vi "ezAFM Practice 1.7.vi"() -> ()   [LabVIEW 2015]
uses:
  D:/LabVIEW for ezAFM/LV-PGC 2019-05a/Special Equipment/ezAFM/NMI Integration Code/ezCommander.dll
  LabVIEW for ezAFM/LV-PGC 2019-05a/Special Equipment/ezAFM/NMI Integration Code/ezCommander.dll
  <vilib>/userdefined/High Color/IMAQdx.ctl
  LabVIEW for ezAFM/LV-PGC 2019-05a/Universal vi's/Global Variables/Globals-EasyAFM.vi
  Globals.vi
  <vilib>/vision/driver/NI_Vision_Acquisition_Software.lvlib
panel:
  out "Index":dbl
  out "Direction":dbl
  out "Searching":bool
  out "Crosshair Found?":bool
  in  "Search":bool
  out "Total Steps":dbl
  out "Current Steps":dbl
  in  "Camera":enum32{"ezAFM Camera"}(tab)
  out "ezAFM Camera":T1(plugin-control)
  in  "Connection to Scan":string
  in  "Enable Automatic \nRepositioning":bool
  out "Imaging Status":string
  out "Automated Imaging":bool
  in  "Main Menu":enum32{"Navigation", "Scanning"}(tab)
  in  "APPROACH":bool
  in  "RETRACT":bool
  in  "Step Size":dbl
  in  "Angle":dbl
  in  "THETA":bool
  in  "MOVE2CROSSHAIR":bool
  in  "Current Crosshair":string(combo)="00 | 01"
  in  "Target Crosshair":string(combo)="00 | 01"
  in  "Motor Speed":u16(ring)=30000 items=["SLOW"=3300, "MEDIUM"=30000, "FAST"=65000]
  in  "Navigation Buttons":T2
  in  "SEARCH":bool
  in  "Image Resolution":u16(ring)=256 items=["32"=32, "64"=64, "128"=128, "256"=256, "512"=512, "1024"=1024, "2048"=2048]
  in  "SELECT CONNECTIONS":bool
  in  "Initialize Automated Imaging":bool
  out "Connections":string[](array[string])
  out "Sequence":string[](array[string])
  in  "Indicators":enum32{"Indicators"}(tab)
  out "XYZ Motor Position":dbl[](array[numeric]) format="%#_4f"
  out "ezAFM Status":dbl
  out "Approaching":bool
  out "ezAFM Connected":bool
  out "Retracting":bool
  out "Scan":bool caption="Scanning"
  out "Tip Approached?":bool
  in  "RESET":bool
  out "XY Position":dbl[](array[numeric])
  in  "QUIT":bool
  # "Use Arrow Keys to manually\nmove the XY Motor"
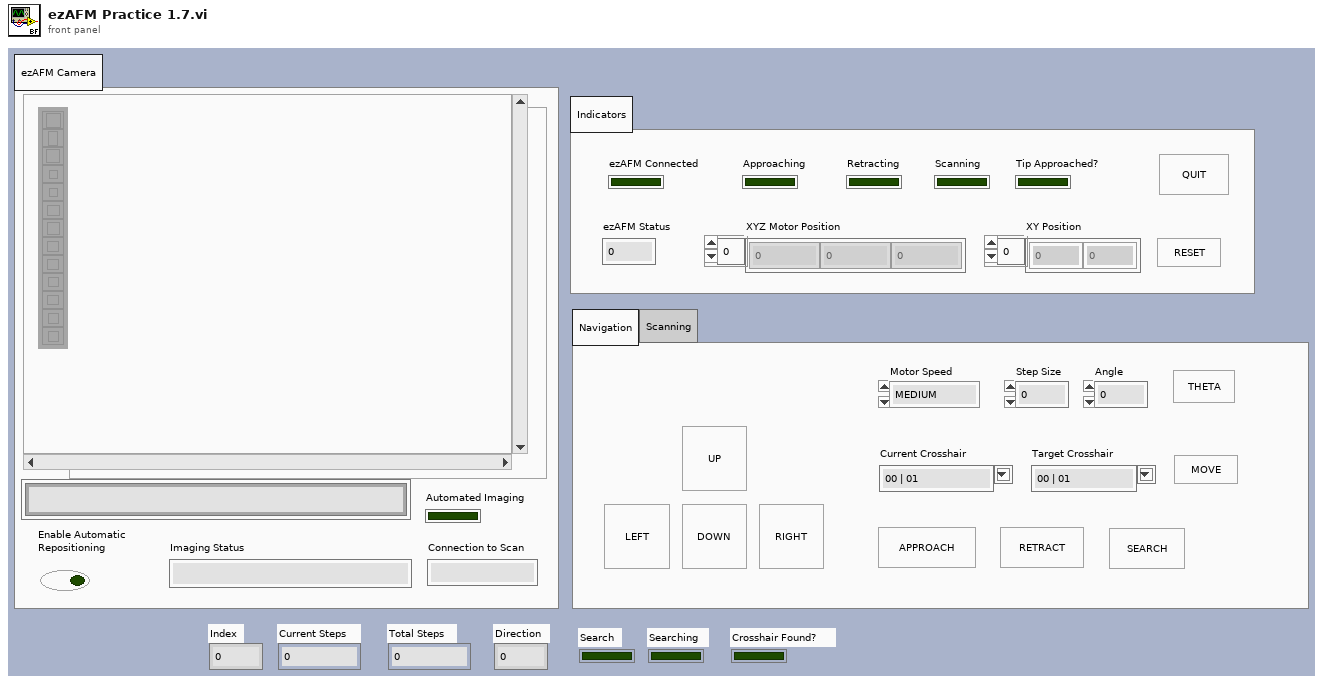
[diagram p1: front panel]
types:
  T1 = typedef "IMAQ Image.ctl" = refnum<image>
  T2 = cluster{"UP":bool, "DOWN":bool, "LEFT":bool, "RIGHT":bool}
  T3 = typedef "IMAQdx.ctl" = refnum<k21>
  T4 = typedef "Image Type" = u32
  T5 = typedef "eventvkey.ctl" = enum16{"ASCII", "Enter", "Return", "Shift", "Ctrl", "Alt", "Cmd", "Opt", "Caps", "NumLock", "Clear", "Break", "Up", "Down", "Left", "Right", "Insert", "Delete", "Home", "End", "PageUp", "PageDown", "Escape", "Help", "Pause", "ScrollLock", "F1", "F2", "F3", "F4", "F5", "F6", "F7", "F8", "F9", "F10", "F11", "F12", "F13", "F14", "F15", "F16", "F17", "F18", "F19", "F20", "F21", "F22", "F23", "F24", "Play", "VolumeUp", "VolumeDown", "Mute", "Two Byte Char"}
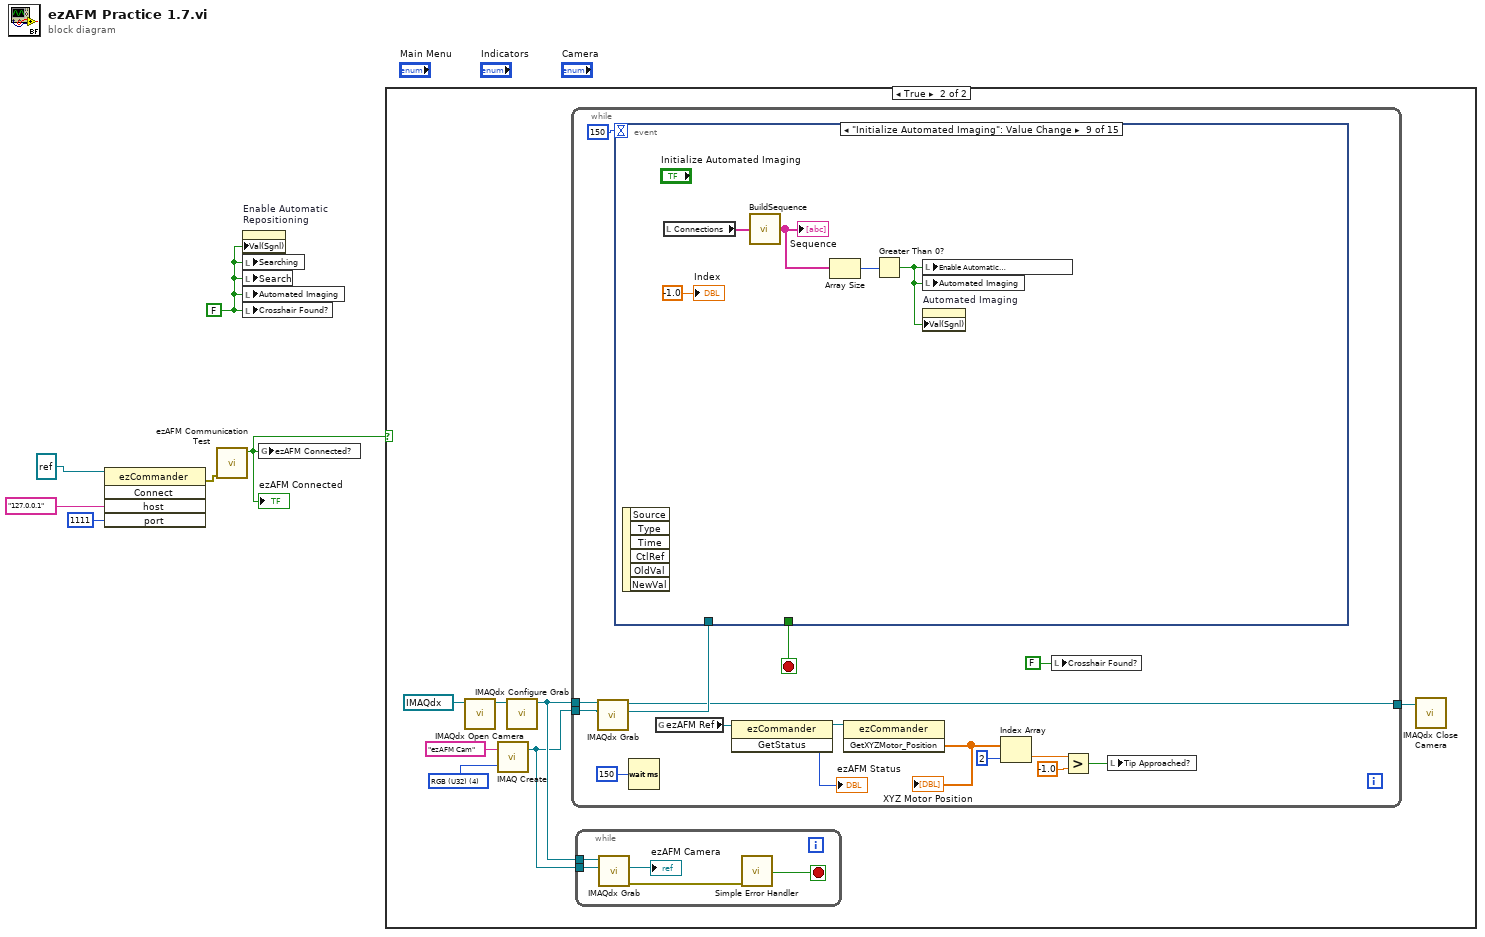
[diagram p0: block diagram]
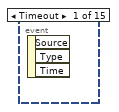
[diagram p3: hidden frame]
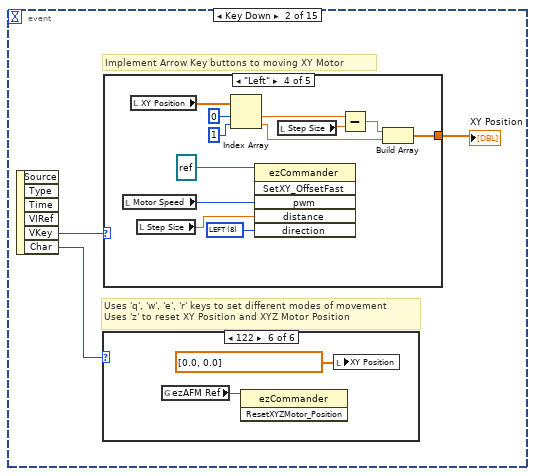
[diagram p4: hidden frame]
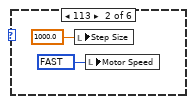
[diagram p6: hidden frame]
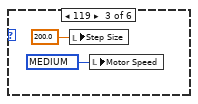
[diagram p7: hidden frame]
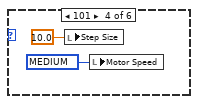
[diagram p8: hidden frame]
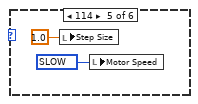
[diagram p9: hidden frame]
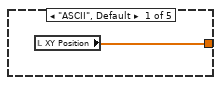
[diagram p10: hidden frame]
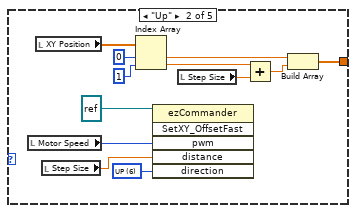
[diagram p11: hidden frame]
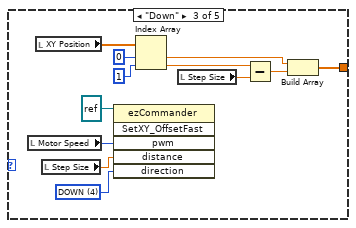
[diagram p12: hidden frame]
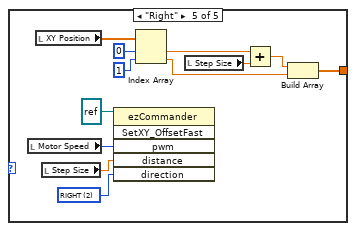
[diagram p13: hidden frame]
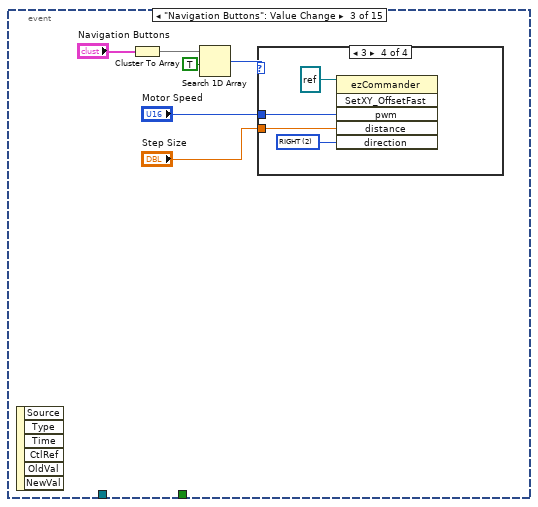
[diagram p14: hidden frame]
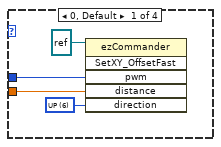
[diagram p15: hidden frame]
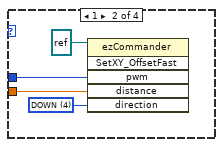
[diagram p16: hidden frame]
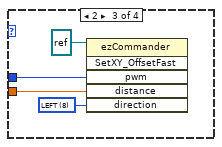
[diagram p17: hidden frame]
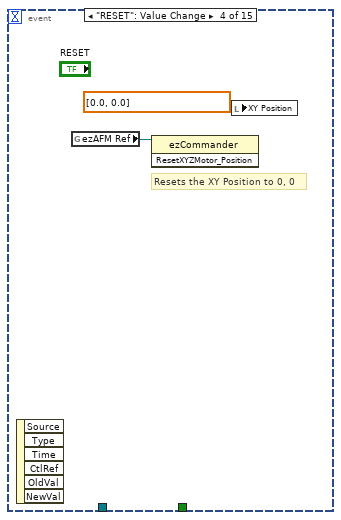
[diagram p18: hidden frame]
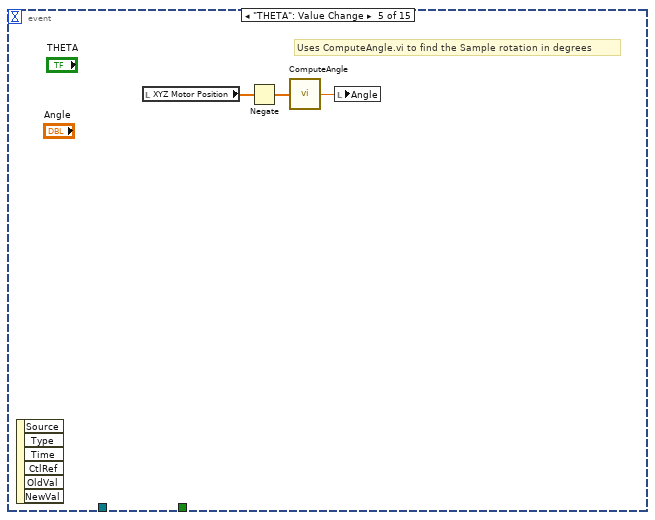
[diagram p19: hidden frame]
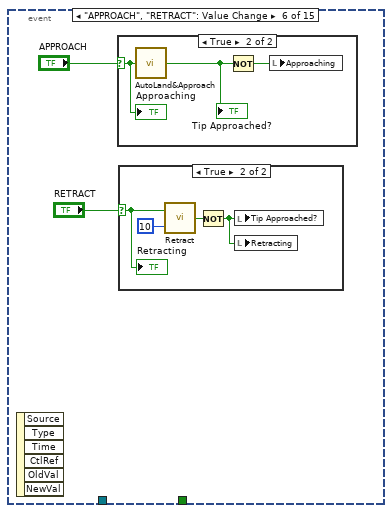
[diagram p20: hidden frame]
diagram:
  w1 = FALSE ("Automated Imaging")
  n1 = invoke class="ezCommander" method="Connect"(reference=refnum<k24> refnum ("ezAFM Ref"), "host"="127.0.0.1", "port"=1111) -> (error out=w5:errorcluster)  [unwired: 2 in, 4 out]
  n2 = call "ezAFM Communication Test.vi"("error in"=w5) -> ("ezAFM COM status"=w2:bool)  [unwired: 3 in, 3 out]
  "ezAFM Connected" <- w2
  n3 = property on="Enable Automatic \nRepositioning" class="Bool (strict)"("Val(Sgnl)"=w1) -> ()  [unwired: 2 in, 2 out]
  n4 = local write "Searching"(w1) -> ()
  n5 = local write "Search"(w1) -> ()
  n6 = local write "Automated Imaging"(w1) -> ()
  n7 = local write "Crosshair Found?"(w1) -> ()
  n8 = global write "Globals.vi" "ezAFM Connected?"(w2) -> ()
  n9 = case shown="True" w2 {
    frame False {
    }
    frame True {
      w10 = T4 4 items=["Grayscale (U8)", "Grayscale (I16)", "Grayscale (SGL)", "Complex (CSG)", "RGB (U32)", "HSL (U32)", "RGB (U64)", "Grayscale (U16)"] ("Image Type")
      n10 = call <vilib>:"IMAQdx Open Camera.vi"("Session In"=T3 "cam5") -> ("Session Out"=w11:T3)  [unwired: 9 in, 1 out]
      n11 = call "IMAQ Create"("Image Name"="ezAFM Cam", "Image Type"=w10) -> ("New Image"=w8:T1)  [unwired: 3 in, 1 out]
      n12 = call <vilib>:"IMAQdx Configure Grab.vi"("Session In"=w11) -> ("Session Out"=w9:T3)  [unwired: 9 in, 1 out]
      n13 = while {
        tunnel: w9 -> [w24]
        tunnel: w8 -> [w23]
        tunnel: [w21] -> w7
        stop <- w20 stop-if-true
        n14 = call <vilib>:"IMAQdx Grab.vi"("Image In"=w23, "Session In"=w24) -> ("Image Out"=w22:T1, "Session Out"=w21:T3)  [unwired: 2 in, 6 out]
        n15 = event shown="[8] \"Initialize Automated Imaging\": Value Change" {
          selector: _ -> [_ _ _ _ _ _ _ _ _ _ _ _ _ _ _]
          dyn-events: _ -> [_ _ _ _ _ _ _ _ _ _ _ _ _ _ _]
          timeout: 150 -> [_ _ _ _ _ _ _ _ _ _ _ _ _ _ _]
          tunnel: [_ _ _ _ _ _ _ _ _ _ _ _ _ _ "QUIT"] -> w20
          tunnel: w22 -> [_ _ _ _ _ _ _ _ _ _ _ _ w188 _ _]
          event Timeout {
            n16 = event-data() -> ()  [unwired: 1 in, 3 out]
          }
          event Key Down {
            # "Uses 'q', 'w', 'e', 'r' keys to set different modes of movement\nUses 'z' to reset XY Position and XYZ Motor Position"
            # "Implement Arrow Key buttons to moving XY Motor"
            n17 = event-data() -> ("VKey"=w35:T5, "Char"=w36:i16)  [unwired: 1 in, 4 out]
            n18 = case shown="122" w36 {
              frame 0, Default {
              }
              frame 113 {
                w38 = u16 65000 items=["SLOW"=3300, "MEDIUM"=30000, "FAST"=65000] ("Motor Speed")
                n19 = local write "Step Size"(1000.0 ("Step Size")) -> ()
                n20 = local write "Motor Speed"(w38) -> ()
              }
              frame 119 {
                w40 = u16 30000 items=["SLOW"=3300, "MEDIUM"=30000, "FAST"=65000] ("Motor Speed")
                n21 = local write "Step Size"(200.0 ("Step Size")) -> ()
                n22 = local write "Motor Speed"(w40) -> ()
              }
              frame 101 {
                w42 = u16 30000 items=["SLOW"=3300, "MEDIUM"=30000, "FAST"=65000] ("Motor Speed")
                n23 = local write "Step Size"(10.0 ("Step Size")) -> ()
                n24 = local write "Motor Speed"(w42) -> ()
              }
              frame 114 {
                w44 = u16 3300 items=["SLOW"=3300, "MEDIUM"=30000, "FAST"=65000] ("Motor Speed")
                n25 = local write "Step Size"(1.0 ("Step Size")) -> ()
                n26 = local write "Motor Speed"(w44) -> ()
              }
              frame 122 {
                n27 = global read "Globals-EasyAFM.vi" "ezAFM Ref"() -> (w46:refnum<k24>)
                n28 = invoke class="ezCommander" method="ResetXYZMotor_Position"(reference=w46) -> ()  [unwired: 2 in, 3 out]
                n29 = local write "XY Position"(dbl[] [0.0, 0.0] ("XY Position")) -> ()
              }
            }
            n30 = case shown="\"Left\"" w35 {
              tunnel: [w48 w50 w61 w73 w85] -> w37
              frame "ASCII", Default {
                n31 = local read "XY Position"() -> (w48:dbl[])
              }
              frame "Up" {
                w59 = u16 6 items=["UP"=6, "DOWN"=4, "LEFT"=8, "RIGHT"=2]
                n32 = local read "Motor Speed"() -> (w58:u16)
                n33 = local read "XY Position"() -> (w56:dbl[])
                n34 = local read "Step Size"() -> (w57:dbl)
                n35 = Index Array(array=w56, index #1=0 ("index"), index #2=1 ("index")) -> (element #1=w52:dbl, element #2=w49:dbl)
                n36 = invoke class="ezCommander" method="SetXY_OffsetFast"(reference=refnum<k24> refnum ("ezAFM Ref"), "pwm"=w58, "distance"=w57, "direction"=w59) -> ()  [unwired: 2 in, 6 out]
                n37 = local read "Step Size"() -> (w53:dbl)
                n38 = Add(x=w49, y=w53) -> (x+y=w51:dbl)
                n39 = Build Array(w52, w51) -> (w50:dbl[])
              }
              frame "Down" {
                w69 = u16 4 items=["UP"=6, "DOWN"=4, "LEFT"=8, "RIGHT"=2]
                n40 = local read "Motor Speed"() -> (w71:u16)
                n41 = local read "XY Position"() -> (w63:dbl[])
                n42 = local read "Step Size"() -> (w70:dbl)
                n43 = invoke class="ezCommander" method="SetXY_OffsetFast"(reference=refnum<k24> refnum ("ezAFM Ref"), "pwm"=w71, "distance"=w70, "direction"=w69) -> ()  [unwired: 2 in, 6 out]
                n44 = Index Array(array=w63, index #1=0 ("index"), index #2=1 ("index")) -> (element #1=w65:dbl, element #2=w66:dbl)
                n45 = local read "Step Size"() -> (w62:dbl)
                n46 = Subtract(x=w66, y=w62) -> (x-y=w64:dbl)
                n47 = Build Array(w65, w64) -> (w61:dbl[])
              }
              frame "Left" {
                w83 = u16 8 items=["UP"=6, "DOWN"=4, "LEFT"=8, "RIGHT"=2]
                n48 = local read "Motor Speed"() -> (w81:u16)
                n49 = local read "XY Position"() -> (w77:dbl[])
                n50 = local read "Step Size"() -> (w82:dbl)
                n51 = Index Array(array=w77, index #1=0 ("index"), index #2=1 ("index")) -> (element #1=w76:dbl, element #2=w74:dbl)
                n52 = invoke class="ezCommander" method="SetXY_OffsetFast"(reference=refnum<k24> refnum ("ezAFM Ref"), "pwm"=w81, "distance"=w82, "direction"=w83) -> ()  [unwired: 2 in, 6 out]
                n53 = local read "Step Size"() -> (w78:dbl)
                n54 = Subtract(x=w76, y=w78) -> (x-y=w75:dbl)
                n55 = Build Array(w75, w74) -> (w73:dbl[])
              }
              frame "Right" {
                w95 = u16 2 items=["UP"=6, "DOWN"=4, "LEFT"=8, "RIGHT"=2]
                n56 = local read "Motor Speed"() -> (w94:u16)
                n57 = local read "XY Position"() -> (w90:dbl[])
                n58 = local read "Step Size"() -> (w93:dbl)
                n59 = invoke class="ezCommander" method="SetXY_OffsetFast"(reference=refnum<k24> refnum ("ezAFM Ref"), "pwm"=w94, "distance"=w93, "direction"=w95) -> ()  [unwired: 2 in, 6 out]
                n60 = Index Array(array=w90, index #1=0 ("index"), index #2=1 ("index")) -> (element #1=w88:dbl, element #2=w86:dbl)
                n61 = local read "Step Size"() -> (w89:dbl)
                n62 = Add(x=w88, y=w89) -> (x+y=w87:dbl)
                n63 = Build Array(w87, w86) -> (w85:dbl[])
              }
            }
            "XY Position" <- w37
          }
          event "Navigation Buttons": Value Change {
            n64 = event-data() -> ()  [unwired: 1 in, 6 out]
            n65 = Cluster To Array(cluster="Navigation Buttons") -> (array=w101:bool[])
            n66 = Search 1D Array(1D array=w101, element=TRUE) -> (index of element=w99:i32)  [unwired: 1 in]
            n67 = case shown="3" w99 {
              tunnel: "Step Size" -> [w103 w108 w112 w116]
              tunnel: "Motor Speed" -> [w104 w107 w111 w115]
              frame 0, Default {
                w105 = u16 6 items=["UP"=6, "DOWN"=4, "LEFT"=8, "RIGHT"=2]
                n68 = invoke class="ezCommander" method="SetXY_OffsetFast"(reference=refnum<k24> refnum ("ezAFM Ref"), "pwm"=w104, "distance"=w103, "direction"=w105) -> ()  [unwired: 2 in, 6 out]
              }
              frame 1 {
                w109 = u16 4 items=["UP"=6, "DOWN"=4, "LEFT"=8, "RIGHT"=2]
                n69 = invoke class="ezCommander" method="SetXY_OffsetFast"(reference=refnum<k24> refnum ("ezAFM Ref"), "pwm"=w107, "distance"=w108, "direction"=w109) -> ()  [unwired: 2 in, 6 out]
              }
              frame 2 {
                w113 = u16 8 items=["UP"=6, "DOWN"=4, "LEFT"=8, "RIGHT"=2]
                n70 = invoke class="ezCommander" method="SetXY_OffsetFast"(reference=refnum<k24> refnum ("ezAFM Ref"), "pwm"=w111, "distance"=w112, "direction"=w113) -> ()  [unwired: 2 in, 6 out]
              }
              frame 3 {
                w117 = u16 2 items=["UP"=6, "DOWN"=4, "LEFT"=8, "RIGHT"=2]
                n71 = invoke class="ezCommander" method="SetXY_OffsetFast"(reference=refnum<k24> refnum ("ezAFM Ref"), "pwm"=w115, "distance"=w116, "direction"=w117) -> ()  [unwired: 2 in, 6 out]
              }
            }
          }
          event "RESET": Value Change {
            # "Resets the XY Position to 0, 0"
            n72 = event-data() -> ()  [unwired: 1 in, 6 out]
            n73 = global read "Globals-EasyAFM.vi" "ezAFM Ref"() -> (w119:refnum<k24>)
            n74 = invoke class="ezCommander" method="ResetXYZMotor_Position"(reference=w119) -> ()  [unwired: 2 in, 3 out]
            n75 = local write "XY Position"(dbl[] [0.0, 0.0] ("XY Position")) -> ()
          }
          event "THETA": Value Change {
            # "Uses ComputeAngle.vi to find the Sample rotation in degrees"
            n76 = event-data() -> ()  [unwired: 1 in, 6 out]
            n77 = local read "XYZ Motor Position"() -> (w122:dbl[])
            n78 = Negate(x=w122) -> (-x=w123:dbl[])
            n79 = call "ComputeAngle.vi"("XY Vector"=w123) -> ("Angle"=w121:dbl)
            n80 = local write "Angle"(w121) -> ()
          }
          event "APPROACH", "RETRACT": Value Change {
            n81 = event-data() -> ()  [unwired: 1 in, 6 out]
            n82 = case shown="True" "APPROACH" {
              selector: "APPROACH" -> [_ w131]
              frame False {
              }
              frame True {
                n83 = call "AutoLand&Approach.vi"("Approaching?"=w131) -> ("Finished?"=w130:bool)
                "Tip Approached?" <- w130
                n84 = Not(x=w130) -> (.not. x?=w132:bool)
                n85 = local write "Approaching"(w132) -> ()
                "Approaching" <- w131
              }
            }
            n86 = case shown="True" "RETRACT" {
              selector: "RETRACT" -> [_ w126]
              frame False {
              }
              frame True {
                n87 = call "Retract.vi"("Number of Cycles"=10, "Retracting?"=w126) -> ("Finished?"=w128:bool)
                n88 = Not(x=w128) -> (.not. x?=w127:bool)
                n89 = local write "Tip Approached?"(w127) -> ()
                n90 = local write "Retracting"(w127) -> ()
                "Retracting" <- w126
              }
            }
          }
          event "MOVE2CROSSHAIR": Value Change {
            w138 = u16 65000 items=["SLOW"=3300, "MEDIUM"=30000, "FAST"=65000] ("Motor Speed")
            # "XY Vector is in cartesian coordinates of the Oasis Camera\nUses Move2Device.vi to find the XY Vector between the Current Device and Target Device crosshairs\nInputs the XY Vector into Move2Vector.vi to command the XY Motor to move"
            n91 = event-data() -> ()  [unwired: 1 in, 6 out]
            n92 = call "GetCrosshairVector.vi"("Target Crosshair"="Target Crosshair", "Current Crosshair"="Current Crosshair") -> ("XY Vector"=w133:dbl[])  [unwired: 9 in]
            n93 = local read "Angle"() -> (w137:dbl)
            n94 = call "Move2Vector.vi"("Motor Speed"=w138, "Angle"=w137, "XY Vector"=w133) -> ("Finished?"=w136:bool)  [unwired: 8 in]
            n95 = case shown="True" w136 {
              frame False {
              }
              frame True {
                n96 = local read "Enable Automatic \nRepositioning"() -> (w141:bool)
                n97 = local read "Target Crosshair"() -> (w140:string)
                n98 = local write "MOVE2CROSSHAIR"(FALSE) -> ()
                n99 = local write "Current Crosshair"(w140) -> ()
                n100 = case shown="True" w141 {
                  frame False {
                  }
                  frame True {
                    n101 = property on="Search" class="Bool (strict)"("Val(Sgnl)"=TRUE ("Value (Signaling)")) -> ()  [unwired: 2 in, 2 out]
                  }
                }
              }
            }
          }
          event "SELECT CONNECTIONS": Value Change {
            n102 = event-data() -> ()  [unwired: 1 in, 6 out]
            n103 = case shown="True" "SELECT CONNECTIONS" {
              frame False {
              }
              frame True {
                n104 = call "SelectConnections.vi"() -> ("Selected Connections"=→"Connections":string[])  [unwired: 1 in]
              }
            }
          }
          event "Initialize Automated Imaging": Value Change {
            n105 = event-data() -> ()  [unwired: 1 in, 6 out]
            n106 = local read "Connections"() -> (w149:string[])
            n107 = call "BuildSequence.vi"("Connections"=w149) -> ("Sequence"=w147:string[])
            "Sequence" <- w147
            n108 = Array Size(array=w147) -> (size(s)=w146:i32)
            n109 = Greater Than 0?(x=w146) -> (x > 0?=w145:bool)
            n110 = local write "Enable Automatic \nRepositioning"(w145) -> ()
            n111 = local write "Automated Imaging"(w145) -> ()
            n112 = property on="Automated Imaging" class="Bool (strict)"("Val(Sgnl)"=w145) -> ()  [unwired: 2 in, 2 out]
            "Index" <- -1.0 ("Index")
          }
          event "Automated Imaging": Value Change {
            n113 = event-data() -> ()  [unwired: 1 in, 6 out]
            n114 = local read "Index"() -> (w154:dbl)
            n115 = local read "Sequence"() -> (w152:string[])
            n116 = Increment(x=w154) -> (x+1=w153:dbl)
            n117 = local write "Index"(w153) -> ()
            n118 = Index Array(array=w152, index=w153) -> (element=w151:string)
            "Imaging Status" <- w151
            n119 = Search/Split String(string=w151, search string/char (-)="Scan Spot") -> (offset of match=w157:i32)  [unwired: 1 in, 2 out]
            n120 = Search/Split String(string=w151, search string/char (-)="Crosshairs") -> (offset of match=w158:i32)  [unwired: 1 in, 2 out]
            n121 = Greater Or Equal To 0?(x=w157) -> (x >= 0?=w156:bool)
            n122 = Greater Or Equal To 0?(x=w158) -> (x >= 0?=w155:bool)
            n123 = case shown="True" w155 {
              tunnel: w151 -> [_ w168]
              frame False {
              }
              frame True {
                n124 = String Subset(string=w168, offset (0)=21, length (rest)=7 ("length (rest)")) -> (substring=w162:string)
                n125 = String Subset(string=w168, offset (0)=10, length (rest)=7 ("length (rest)")) -> (substring=w163:string)
                n126 = local write "Current Crosshair"(w163) -> ()
                n127 = local write "Target Crosshair"(w162) -> ()
                n128 = String Length(string=w163) -> (length=w164:i32)
                n129 = String Length(string=w162) -> (length=w165:i32)
                n130 = Greater Than 0?(x=w164) -> (x > 0?=w166:bool)
                n131 = Greater Than 0?(x=w165) -> (x > 0?=w167:bool)
                n132 = And(x=w166, y=w167) -> (x .and. y?=w161:bool)
                n133 = property on="MOVE2CROSSHAIR" class="Bool (strict)"("Val(Sgnl)"=w161) -> ()  [unwired: 2 in, 2 out]
              }
            }
            n134 = case shown="True" w156 {
              tunnel: w151 -> [_ w177]
              frame False {
              }
              frame True {
                n135 = String Subset(string=w177, offset (0)=25) -> (substring=w174:string)  [unwired: 1 in]
                n136 = local write "Connection to Scan"(w174) -> ()
                n137 = String Length(string=w174) -> (length=w175:i32)
                n138 = Greater Than 0?(x=w175) -> (x > 0?=w173:bool)
                n139 = property on="Scan" class="Bool (strict)"("Val(Sgnl)"=w173) -> ()  [unwired: 2 in, 2 out]
              }
            }
            n140 = Wait (ms)(milliseconds to wait=u32 1000) -> ()  [unwired: 1 out]
          }
          event "Scan": Value Change {
            n141 = event-data() -> ()  [unwired: 1 in, 6 out]
            n142 = local read "Angle"() -> (w181:dbl)
            n143 = local read "Automated Imaging"() -> (w180:bool)
            n144 = call "TakeScan.vi"("Angle"=w181, "Image Resolution"="Image Resolution", "Connection"="Connection to Scan") -> ("Finished?"=w179:bool)  [unwired: 8 in]
            n145 = And(x=w179, y=w180) -> (x .and. y?=w178:bool)
            n146 = case shown="True" w178 {
              frame False {
              }
              frame True {
                n147 = property on="Automated Imaging" class="Bool (strict)"("Val(Sgnl)"=TRUE ("Value (Signaling)")) -> ()  [unwired: 2 in, 2 out]
              }
            }
          }
          event "Enable Automatic \nRepositioning": Value Change {
            w185 = u16 6 items=["UP"=6, "DOWN"=4, "LEFT"=8, "RIGHT"=2]
            n148 = event-data() -> ()  [unwired: 1 in, 6 out]
            "Total Steps" <- 1.0 ("Total Distance")
            "Current Steps" <- 0.0 ("Current Steps")
            "Direction" <- w185
          }
          event "SEARCH", "Search": Value Change {
            n149 = event-data() -> ("NewVal"=w189:bool)  [unwired: 1 in, 5 out]
            n150 = while {
              tunnel: w188 -> [w198]
              tunnel: [w194] -> w190
              tunnel: [w197] -> w191
              i -> [w195]
              stop <- w192 stop-if-true
              n151 = Greater?(x=w195, y=5.0) -> (0:w193:bool)
              n152 = call "IdentifyCrosshair.vi"("ezAFM Camera"=w198) -> ("Delta"=w197:dbl[], "Found?"=w194:bool)
              n153 = Or(x=w193, y=w194) -> (x .or. y?=w192:bool)
            }
            "Crosshair Found?" <- w190
            n154 = local write "Searching"(w189) -> ()
            n155 = case shown="True" w190 {
              tunnel: w191 -> [_ w209]
              frame False {
                n156 = local read "Enable Automatic \nRepositioning"() -> (w200:bool)
                n157 = local write "Searching"(FALSE ("Searching")) -> ()
                n158 = case shown="True" w200 {
                  frame False {
                  }
                  frame True {
                    n159 = property on="Searching" class="Bool (strict)"("Val(Sgnl)"=TRUE ("Value (Signaling)")) -> ()  [unwired: 2 in, 2 out]
                  }
                }
              }
              frame True {
                w207 = FALSE ("SEARCH")
                w208 = u16 3300 items=["SLOW"=3300, "MEDIUM"=30000, "FAST"=65000] ("Motor Speed")
                n160 = local write "Search"(w207) -> ()
                n161 = local write "Searching"(w207) -> ()
                n162 = call "Move2Vector.vi"("Motor Speed"=w208, "Angle"=0.0, "XY Vector"=w209) -> ("Finished?"=w202:bool)  [unwired: 8 in]
                n163 = local read "Automated Imaging"() -> (w204:bool)
                n164 = property on="Enable Automatic \nRepositioning" class="Bool (strict)"("Val(Sgnl)"=TRUE ("Value (Signaling)")) -> ()  [unwired: 2 in, 2 out]
                n165 = And(x=w204, y=w202) -> (x .and. y?=w203:bool)
                n166 = case shown="True" w203 {
                  selector: w203 -> [_ w210]
                  frame False {
                  }
                  frame True {
                    n167 = property on="Automated Imaging" class="Bool (strict)"("Val(Sgnl)"=w210) -> ()  [unwired: 2 in, 2 out]
                  }
                }
              }
            }
          }
          event "Searching": Value Change {
            n168 = event-data() -> ()  [unwired: 1 in, 6 out]
            n169 = local read "Total Steps"() -> (w213:dbl)
            n170 = local read "Current Steps"() -> (w214:dbl)
            n171 = local read "Direction"() -> (w215:dbl)
            n172 = Equal?(x=w213, y=w214) -> (x = y?=w216:bool)
            n173 = case shown="False" w216 {
              tunnel: w214 -> [w221 _]
              tunnel: w215 -> [w222 w231]
              tunnel: w213 -> [w217 w227]
              tunnel: [TRUE ("Value (Signaling)") TRUE ("Value (Signaling)")] -> w212
              tunnel: [w217 w226] -> w211
              frame False {
                w223 = u16 65000 items=["SLOW"=3300, "MEDIUM"=30000, "FAST"=65000] ("Motor Speed")
                n174 = Increment(x=w221) -> (x+1=w220:dbl)
                n175 = local write "Current Steps"(w220) -> ()
                n176 = invoke class="ezCommander" method="SetXY_OffsetFast"(reference=refnum<k24> refnum ("ezAFM Ref"), "pwm"=w223, "distance"=20.0, "direction"=w222) -> ()  [unwired: 2 in, 6 out]
                n177 = Wait (ms)(milliseconds to wait=u32 500) -> ()  [unwired: 1 out]
              }
              frame True {
                n178 = case shown="6" w231 {
                  tunnel: [u16 0 w234 w235 w236 w237] -> w230
                  frame Default {
                  }
                  frame 6 {
                    w234 = u16 2 items=["UP"=6, "DOWN"=4, "LEFT"=8, "RIGHT"=2]
                  }
                  frame 4 {
                    w235 = u16 8 items=["UP"=6, "DOWN"=4, "LEFT"=8, "RIGHT"=2]
                  }
                  frame 8 {
                    w236 = u16 6 items=["UP"=6, "DOWN"=4, "LEFT"=8, "RIGHT"=2]
                  }
                  frame 2 {
                    w237 = u16 4 items=["UP"=6, "DOWN"=4, "LEFT"=8, "RIGHT"=2]
                  }
                }
                n179 = local write "Current Steps"(0.0 ("Current Steps")) -> ()
                n180 = local write "Direction"(w230) -> ()
                n181 = Increment(x=w227) -> (x+1=w226:dbl)
                n182 = Wait (ms)(milliseconds to wait=u32 500) -> ()  [unwired: 1 out]
              }
            }
            n183 = property on="Search" class="Bool (strict)"("Val(Sgnl)"=w212) -> ()  [unwired: 2 in, 2 out]
            n184 = local write "Total Steps"(w211) -> ()
          }
          event "QUIT": Value Change {
            w239 = FALSE ("ezAFM Connected?")
            n185 = event-data() -> ()  [unwired: 1 in, 6 out]
            n186 = global write "Globals.vi" "ezAFM Connected?"(w239) -> ()
            n187 = local write "ezAFM Connected"(w239) -> ()
          }
        }
        n188 = Wait (ms)(milliseconds to wait=u32 150) -> ()  [unwired: 1 out]
        n189 = global read "Globals-EasyAFM.vi" "ezAFM Ref"() -> (w26:refnum<k24>)
        n190 = invoke class="ezCommander" method="GetStatus"(reference=w26) -> (reference out=w28:refnum<k24>, "GetStatus"=→"ezAFM Status":i32)  [unwired: 2 in, 1 out]
        n191 = invoke class="ezCommander" method="GetXYZMotor_Position"(reference=w28) -> ("GetXYZMotor_Position"=w29:dbl[])  [unwired: 2 in, 2 out]
        "XYZ Motor Position" <- w29
        n192 = Index Array(array=w29, index=2) -> (element=w30:dbl)
        n193 = local write "Crosshair Found?"(FALSE ("Scan")) -> ()
        n194 = Greater?(x=w30, y=-1.0) -> (0:w25:bool)
        n195 = local write "Tip Approached?"(w25) -> ()
      }
      n196 = while {
        tunnel: w9 -> [w18]
        tunnel: w8 -> [w17]
        stop <- w14 stop-if-true
        n197 = call <vilib>:"IMAQdx Grab.vi"("Image In"=w17, "Session In"=w18) -> ("error out"=w15:errorcluster, "Image Out"=→"ezAFM Camera":T1)  [unwired: 2 in, 6 out]
        n198 = call <vilib>:"Simple Error Handler.vi"("error in (no error)"=w15) -> ("error?"=w14:bool)  [unwired: 4 in, 4 out]
      }
      n199 = call <vilib>:"IMAQdx Close Camera.vi"("Session In"=w7) -> ()  [unwired: 10 in, 1 out]
    }
  }
